vi "drop_file_sort.vi"(2 "drop-array":string[](array[string]), 3 "filetypes":string) -> (0 "playlist-array":string[](array[string]), 1 "file-array":string[](array[string]))   [LabVIEW 2012]
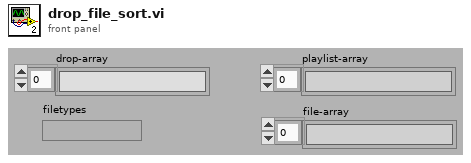
[diagram p1: front panel]
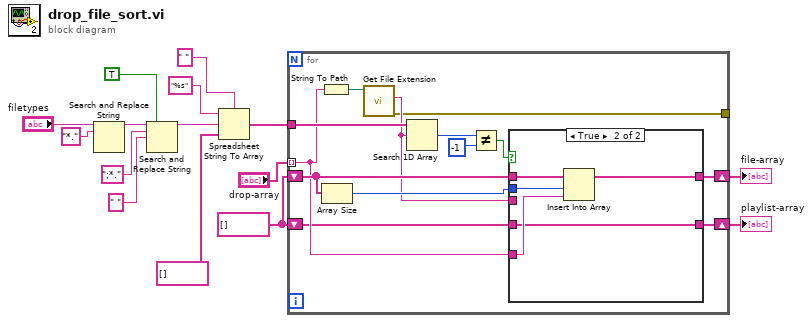
[diagram p0: block diagram]
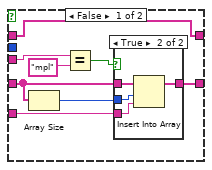
[diagram p2: hidden frame]
diagram:
  w15 = string[] []
  n1 = Search and Replace String(input string="filetypes", search string="*." ("Such-String")) -> (result string=w7:string)  [unwired: 6 in, 3 out]
  n2 = Search and Replace String(replace all?=TRUE ("Alle ersetzen? (F)"), input string=w7, search string=";*." ("Such-String"), replace string=" " ("String ersetzen(\"\")")) -> (result string=w6:string)  [unwired: 4 in, 3 out]
  n3 = Spreadsheet String To Array(delimiter (Tab)=" " ("Trennzeichen (Tabulator)"), format string="%s" ("Format-String"), spreadsheet string=w6, array type (2D Dbl)=string[] []) -> (array=w1:string[])
  n4 = for {
    tunnel: "drop-array" -> [w21] mode=indexing
    shift-right: [w20] -> w12
    shift-left: w15 -> [w23]
    shift-right: [w17] -> w14
    shift-left: w15 -> [w18]
    tunnel: w1 -> [w25]
    tunnel: [w16] -> _
    n5 = String To Path(string=w21) -> (path=w28:path)
    n6 = Array Size(array=w23) -> (size(s)=w22:i32)
    n7 = call <vilib>:"Get File Extension.vi"("file"=w28) -> ("error out"=w16:errorcluster, "lowercase file extension"=w19:string)  [unwired: 7 in, 2 out]
    n8 = Search 1D Array(1D array=w25, element=w19) -> (index of element=w27:i32)  [unwired: 1 in]
    n9 = Not Equal?(x=w27, y=-1) -> (x != y?=w24:bool)
    n10 = case shown="True" w24 {
      tunnel: w23 -> [w36 w46]
      tunnel: w22 -> [_ w45]
      tunnel: w21 -> [w29 w44]
      tunnel: [w36 w43] -> w20
      tunnel: w19 -> [w31 _]
      tunnel: w18 -> [w32 w42]
      tunnel: [w30 w42] -> w17
      frame False {
        n11 = Array Size(array=w32) -> (size(s)=w33:i32)
        n12 = Equal?(x=w31, y="mpl") -> (x = y?=w34:bool)
        n13 = case shown="True" w34 {
          tunnel: w33 -> [_ w41]
          tunnel: w32 -> [w37 w40]
          tunnel: w29 -> [_ w39]
          tunnel: [w37 w38] -> w30
          frame False {
          }
          frame True {
            n14 = Insert Into Array(array=w40, index=w41, new element=w39) -> (w38:string[])
          }
        }
      }
      frame True {
        n15 = Insert Into Array(array=w46, index=w45, new element=w44) -> (w43:string[])
      }
    }
  }
  "playlist-array" <- w14
  "file-array" <- w12
